vi "Delete the Schema.vi"(8 "error in (no error)":errorcluster, 11 "Post Analysis in":refnum<class "Post Analysis.lvclass">) -> (0 "error out":errorcluster, 3 "Post Analysis out":refnum<class "Post Analysis.lvclass">)   [LabVIEW 2023, in "Data Analysis.lvlib" / "Post Analysis.lvlib" / "Post Analysis.lvclass"]
uses:
  Post Analysis.lvclass
  Post Analysis.lvclass/Post Analysis.ctl
  HardwareAbstractionLayer_LVOOP/Database/Database.lvclass
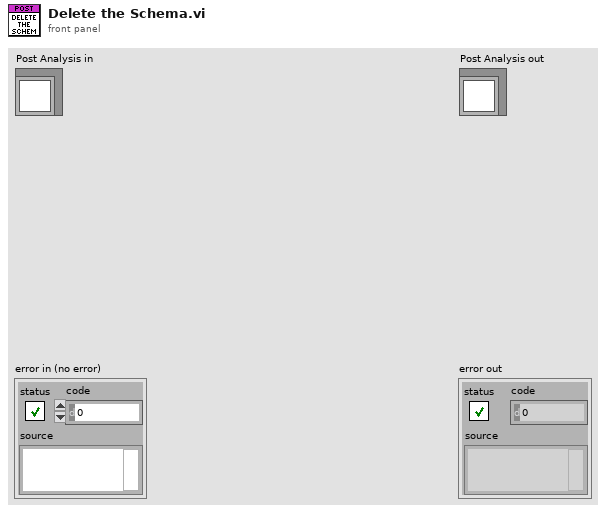
[diagram p1: front panel]
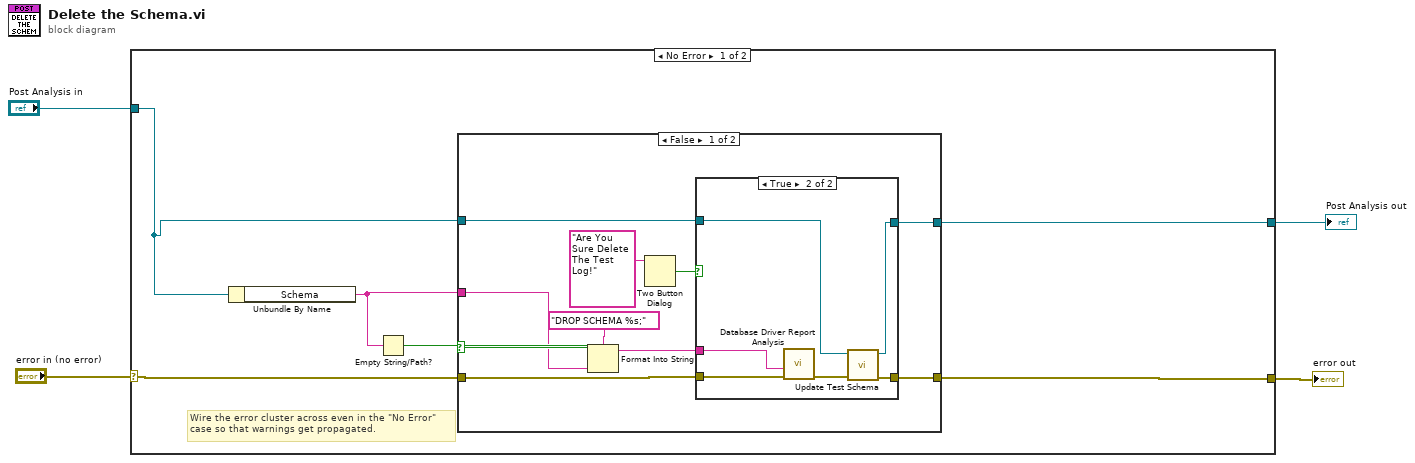
[diagram p0: block diagram]
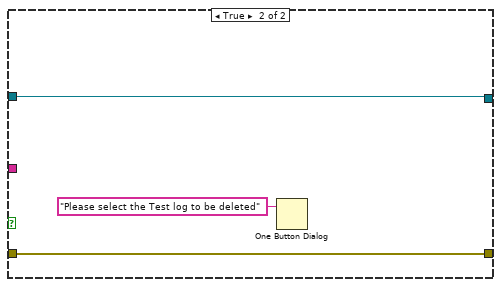
[diagram p3: hidden frame]
diagram:
  n1 = case shown="No Error" "error in (no error)" {
    selector: "error in (no error)" -> [w10 w32]
    tunnel: [w9 w32] -> w3
    tunnel: [w5 w31] -> w1
    tunnel: "Post Analysis in" -> [w6 w31]
    frame No Error {
      # "Wire the error cluster across even in the \"No Error\"\ncase so that warnings get propagated."
      n2 = Unbundle By Name(w6) -> ("Schema"=w7:string)
      n3 = Empty String/Path?(string/path=w7) -> (empty?=w8:bool)
      n4 = case shown="False" w8 {
        tunnel: w10 -> [w19 w30]
        tunnel: [w13 w30] -> w9
        tunnel: w7 -> [w14 _]
        tunnel: w6 -> [w12 w28]
        tunnel: [w11 w28] -> w5
        frame False {
          n5 = Format Into String(format string="DROP SCHEMA %s;", w14) -> (resulting string=w15:string)  [unwired: 2 in, 1 out]
          n6 = Two Button Dialog(message="Are You Sure Delete The Test Log!") -> (T button?=w17:bool)  [unwired: 2 in]
          n7 = case shown="True" w17 {
            tunnel: w19 -> [w21 w27]
            tunnel: w15 -> [_ w26]
            tunnel: [w21 w25] -> w13
            tunnel: w12 -> [w20 w23]
            tunnel: [w20 w22] -> w11
            frame False {
            }
            frame True {
              n8 = call "Database Driver Report Analysis.vi"("error in"=w27, "SQL query"=w26) -> ("error out"=w24:errorcluster)  [unwired: 6 in, 3 out]
              n9 = call "Update Test Schema.vi"("error in (no error)"=w24, "Post Analysis in"=w23) -> ("error out"=w25:errorcluster, "Post Analysis out"=w22:refnum<class "Post Analysis.lvclass">)  [unwired: 8 in]
            }
          }
        }
        frame True {
          n10 = One Button Dialog(message="Please select the Test log to be deleted") -> ()  [unwired: 1 in, 1 out]
        }
      }
    }
    frame Error {
    }
  }
  "error out" <- w3
  "Post Analysis out" <- w1
